vi "Create All Message Queues.vi"(8 "error in (no error)":errorcluster) -> (0 "error out":errorcluster, 3 "Message Queues out":T1)   [LabVIEW 2020, in "Message Queue.lvlib"]
doc: "This VI creates and initializes all the message queues for your application. If your application requires more than one message queue, right-click the \"Message Queues\" constant above and select Open Type Def. Add the new Message Queue(s) to the type definition, then initialize them in this VI."
uses:
  Message Queue.lvlib
  All Message Queues.ctl
  Message Cluster.ctl
  Enqueue Message (Single).vi
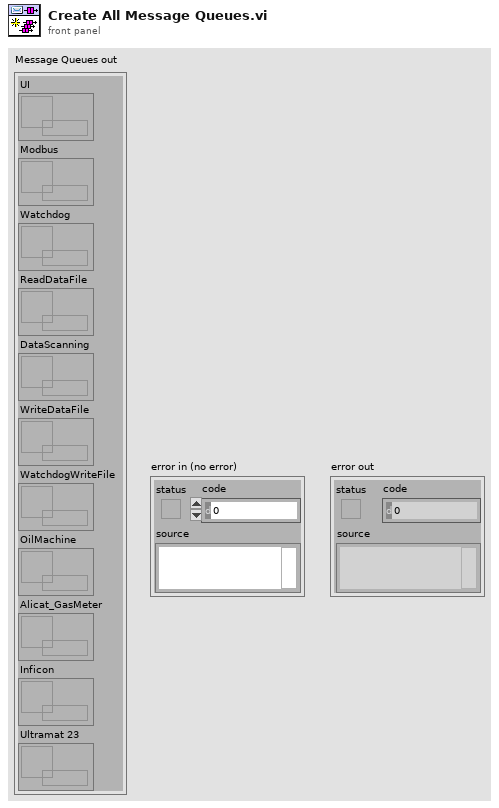
[diagram p1: front panel]
types:
  T1 = typedef "Message Queue.lvlib/All Message Queues.ctl" = cluster{"UI":refnum<queue>, "Modbus":refnum<queue>, "Watchdog":refnum<queue>, "ReadDataFile":refnum<queue>, "DataScanning":refnum<queue>, "WriteDataFile":refnum<queue>, "WatchdogWriteFile":refnum<queue>, "OilMachine":refnum<queue>, "Alicat_GasMeter":refnum<queue>, "Inficon":refnum<queue>, "Ultramat 23":refnum<queue>}
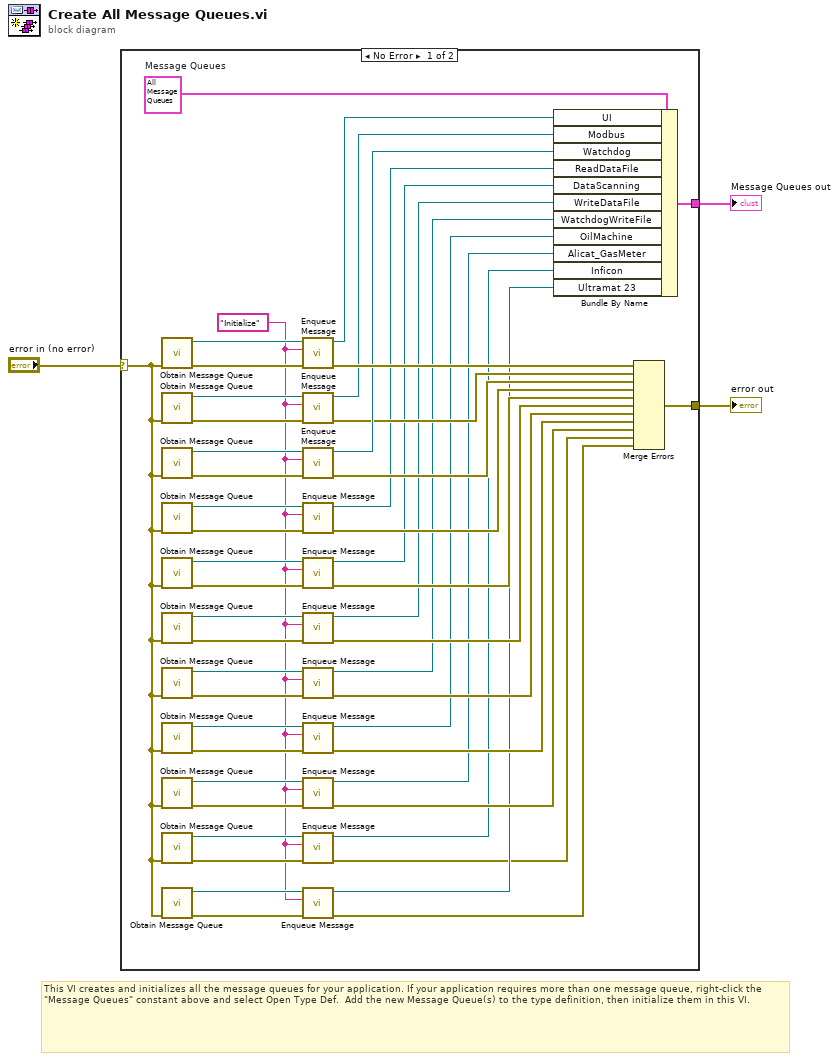
[diagram p0: block diagram]
diagram:
  # "This VI creates and initializes all the message queues for your application. If your application requires more than one message queue, right-click the \"Message Queues\" constant above and select Open Type Def.  Add the new Message Queue(s) to the type definition, then initialize them in this VI."
  n1 = case shown="No Error" "error in (no error)" {
    selector: "error in (no error)" -> [w7 w53]
    tunnel: [w31 w53] -> w3
    tunnel: [w50 _] -> w1
    frame No Error {
      w8 = "Initialize" ("Message")
      w51 = T1 {"UI"=refnum, "Modbus"=refnum, "Watchdog"=refnum, "ReadDataFile"=refnum, "DataScanning"=refnum, "WriteDataFile"=refnum, "WatchdogWriteFile"=refnum, "OilMachine"=refnum, "Alicat_GasMeter"=refnum, "Inficon"=refnum, "Ultramat 23"=refnum}  # Message Queues
      n2 = call "Obtain Message Queue.vi"("error in (no error)"=w7) -> ("error out"=w49:errorcluster, "Message Queue"=w48:refnum<queue>)  [unwired: 9 in]
      n3 = call "Obtain Message Queue.vi"("error in (no error)"=w7) -> ("error out"=w46:errorcluster, "Message Queue"=w47:refnum<queue>)  [unwired: 9 in]
      n4 = call "Obtain Message Queue.vi"("error in (no error)"=w7) -> ("error out"=w45:errorcluster, "Message Queue"=w44:refnum<queue>)  [unwired: 9 in]
      n5 = call "Obtain Message Queue.vi"("error in (no error)"=w7) -> ("error out"=w38:errorcluster, "Message Queue"=w37:refnum<queue>)  [unwired: 9 in]
      n6 = call "Obtain Message Queue.vi"("error in (no error)"=w7) -> ("error out"=w34:errorcluster, "Message Queue"=w33:refnum<queue>)  [unwired: 9 in]
      n7 = call "Obtain Message Queue.vi"("error in (no error)"=w7) -> ("error out"=w29:errorcluster, "Message Queue"=w27:refnum<queue>)  [unwired: 9 in]
      n8 = call "Obtain Message Queue.vi"("error in (no error)"=w7) -> ("error out"=w25:errorcluster, "Message Queue"=w22:refnum<queue>)  [unwired: 9 in]
      n9 = call "Obtain Message Queue.vi"("error in (no error)"=w7) -> ("error out"=w21:errorcluster, "Message Queue"=w18:refnum<queue>)  [unwired: 9 in]
      n10 = call "Obtain Message Queue.vi"("error in (no error)"=w7) -> ("error out"=w16:errorcluster, "Message Queue"=w17:refnum<queue>)  [unwired: 9 in]
      n11 = call "Obtain Message Queue.vi"("error in (no error)"=w7) -> ("error out"=w13:errorcluster, "Message Queue"=w12:refnum<queue>)  [unwired: 9 in]
      n12 = call "Obtain Message Queue.vi"("error in (no error)"=w7) -> ("error out"=w9:errorcluster, "Message Queue"=w10:refnum<queue>)  [unwired: 9 in]
      n13 = call-poly "Enqueue Message.vi"("error in (no error)"=w49, "Message"=w8, "Message Queue"=w48) -> ("error out"=w52:errorcluster, "dup Message Queue"=w43:refnum<queue>)  [unwired: 7 in]
      n14 = call-poly "Enqueue Message.vi"("error in (no error)"=w46, "Message"=w8, "Message Queue"=w47) -> ("error out"=w40:errorcluster, "dup Message Queue"=w42:refnum<queue>)  [unwired: 7 in]
      n15 = call-poly "Enqueue Message.vi"("error in (no error)"=w45, "Message"=w8, "Message Queue"=w44) -> ("error out"=w39:errorcluster, "dup Message Queue"=w41:refnum<queue>)  [unwired: 7 in]
      n16 = call-poly "Enqueue Message.vi"("error in (no error)"=w38, "Message"=w8, "Message Queue"=w37) -> ("error out"=w36:errorcluster, "dup Message Queue"=w35:refnum<queue>)  [unwired: 7 in]
      n17 = call-poly "Enqueue Message.vi"("error in (no error)"=w34, "Message"=w8, "Message Queue"=w33) -> ("error out"=w32:errorcluster, "dup Message Queue"=w30:refnum<queue>)  [unwired: 7 in]
      n18 = call-poly "Enqueue Message.vi"("error in (no error)"=w29, "Message"=w8, "Message Queue"=w27) -> ("error out"=w26:errorcluster, "dup Message Queue"=w28:refnum<queue>)  [unwired: 7 in]
      n19 = call-poly "Enqueue Message.vi"("error in (no error)"=w25, "Message"=w8, "Message Queue"=w22) -> ("error out"=w24:errorcluster, "dup Message Queue"=w23:refnum<queue>)  [unwired: 7 in]
      n20 = call-poly "Enqueue Message.vi"("error in (no error)"=w21, "Message"=w8, "Message Queue"=w18) -> ("error out"=w20:errorcluster, "dup Message Queue"=w19:refnum<queue>)  [unwired: 7 in]
      n21 = call-poly "Enqueue Message.vi"("error in (no error)"=w16, "Message"=w8, "Message Queue"=w17) -> ("error out"=w15:errorcluster, "dup Message Queue"=w14:refnum<queue>)  [unwired: 7 in]
      n22 = call-poly "Enqueue Message.vi"("error in (no error)"=w13, "Message"=w8, "Message Queue"=w12) -> ("error out"=w5:errorcluster, "dup Message Queue"=w11:refnum<queue>)  [unwired: 7 in]
      n23 = call-poly "Enqueue Message.vi"("error in (no error)"=w9, "Message"=w8, "Message Queue"=w10) -> ("error out"=w4:errorcluster, "dup Message Queue"=w6:refnum<queue>)  [unwired: 7 in]
      n24 = Bundle By Name(cluster=w51, "UI"=w43, "Modbus"=w42, "Watchdog"=w41, "ReadDataFile"=w35, "DataScanning"=w30, "WriteDataFile"=w28, "WatchdogWriteFile"=w23, "OilMachine"=w19, "Alicat_GasMeter"=w14, "Inficon"=w11, "Ultramat 23"=w6) -> (w50:T1)
      n25 = Merge Errors(w52, w40, w39, w36, w32, w26, w24, w20, w15, w5, w4) -> (w31:errorcluster)
    }
    frame Error {
    }
  }
  "Message Queues out" <- w1
  "error out" <- w3
